vi "8bit sync-Gen patches montage B.vi"(0 "U8 Image (Montage)":T3, 1 "max value":dbl, 4 "Cycle number":i32, 5 "error in (no error)":errorcluster, 6 "Coordinates of montage positions":cluster{"X\n\nY":i32[]}[](array[cluster]), 8 "Extracted patches AVIs refs":T1[](array[typedef]), 9 "Frames info":T4, 11 "Image refs cluster":T2) -> (16 "U8 Image (Montage)":T3, 19 "error out":errorcluster)   [LabVIEW 2020]
uses:
  <vilib>/vision/Image Controls.llb/IMAQ Image.ctl
  Typedefs/8bit sync-IMAQ image refs.ctl
  <vilib>/vision/Avi.llb/IMAQ AVI2 Refnum.ctl
  Globals/gl_8-bit montage window ctrl refs.vi
  <vilib>/vision/NI_Vision_Development_Module.lvlib
panel:
  out "max value 3":u8
  out "max value 2":dbl
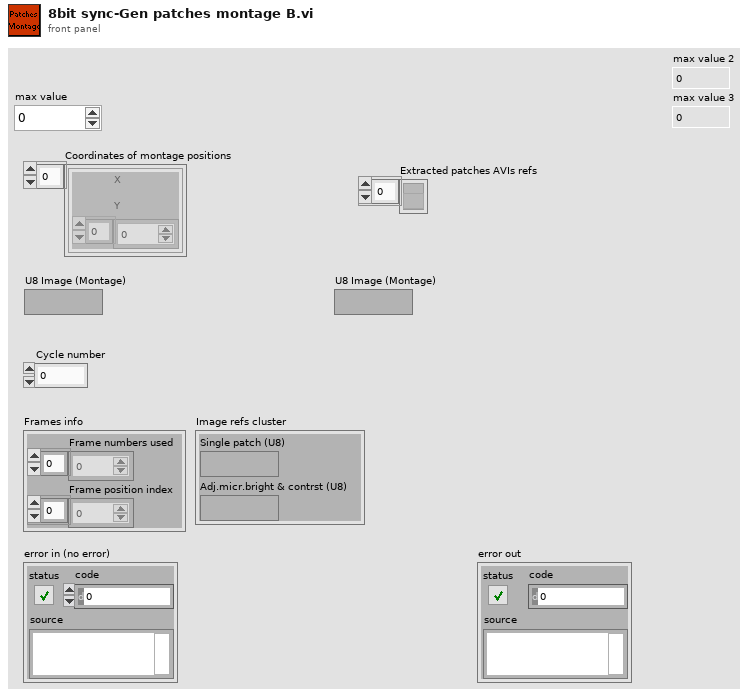
[diagram p1: front panel]
types:
  T1 = typedef "IMAQ AVI2 Refnum.ctl" = refnum<k20>
  T2 = typedef "8bit sync-IMAQ image refs.ctl" = cluster{"Single patch (U8)":T3, "Adj.micr.bright & contrst (U8)":T3}
  T3 = typedef "IMAQ Image.ctl" = refnum<image>
  T4 = cluster{"Frame numbers used":i32[], "Frame position index":i32[]}
  T5 = typedef "Image Type" = u32
  T6 = typedef "8-bit video export window ctrl refs.ctl" = cluster{"This VI":refnum<vi>, "Add speed data":refnum<vi>, "Add camera videos":refnum<vi>, "Stop button":refnum<vi>, "Camera Video Adjustments":refnum<vi>, "Microscope Image Adjustments":refnum<vi>, "Execute":refnum<vi>, "Codec":refnum<vi>, "Channel to load":refnum<vi>, "Speed graph behaviour":refnum<vi>, "Include speed graph":refnum<vi>, "Number of rows to generate":refnum<vi>, "Path":refnum<vi>}
  T7 = typedef "Bright-Contr-Gamma cluster.ctl" = cluster{"Brightness":sgl, "Contrast":sgl, "Gamma":sgl}
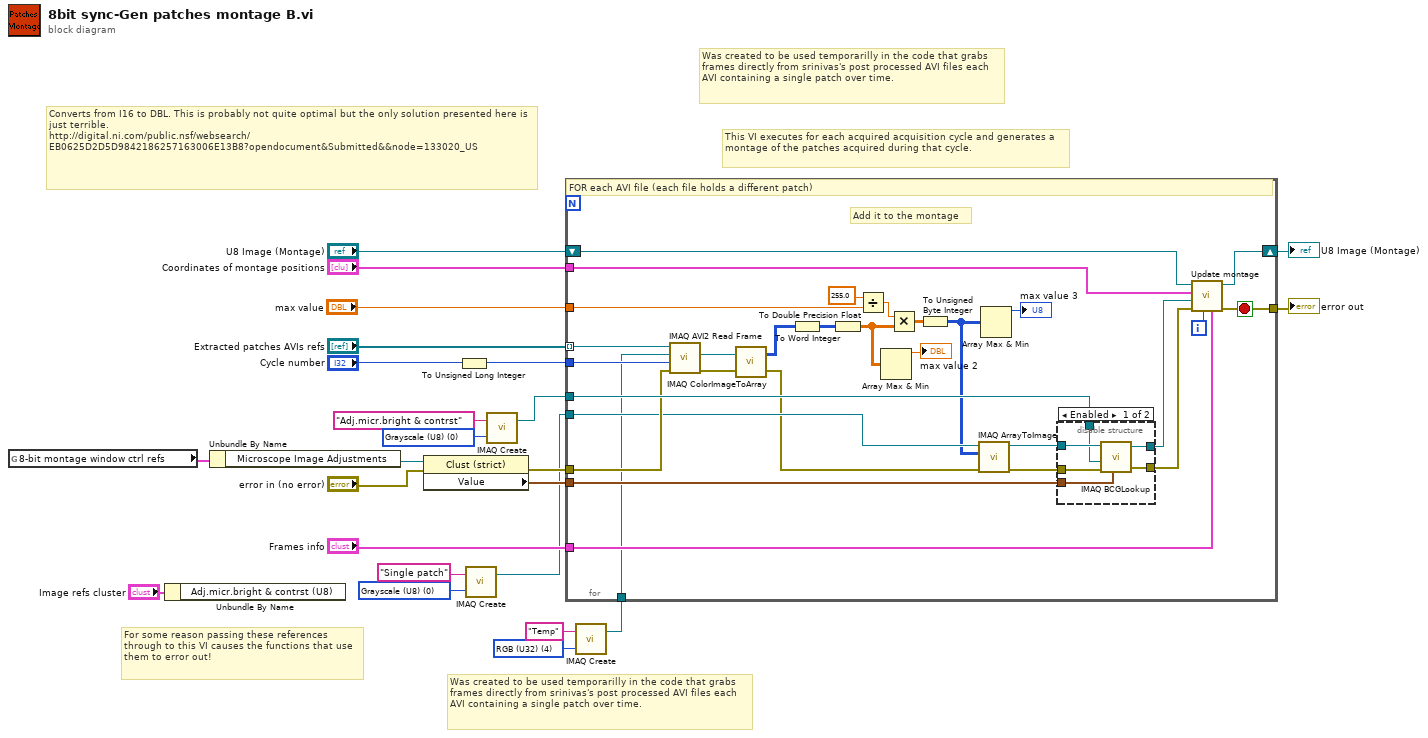
[diagram p0: block diagram]
diagram:
  w3 = T5 0 items=["Grayscale (U8)", "Grayscale (I16)", "Grayscale (SGL)", "Complex (CSG)", "RGB (U32)", "HSL (U32)", "RGB (U64)", "Grayscale (U16)"] ("Image Type")
  w6 = T5 0 items=["Grayscale (U8)", "Grayscale (I16)", "Grayscale (SGL)", "Complex (CSG)", "RGB (U32)", "HSL (U32)", "RGB (U64)", "Grayscale (U16)"] ("Image Type")
  w8 = T5 4 items=["Grayscale (U8)", "Grayscale (I16)", "Grayscale (SGL)", "Complex (CSG)", "RGB (U32)", "HSL (U32)", "RGB (U64)", "Grayscale (U16)"] ("Image Type")
  # "For some reason passing these references through to this VI causes the functions that use them to error out!"
  # "Was created to be used temporarilly in the code that grabs frames directly from srinivas's post processed AVI files each AVI containing a single patch over time."
  # "Was created to be used temporarilly in the code that grabs frames directly from srinivas's post processed AVI files each AVI containing a single patch over time."
  # "Converts from I16 to DBL. This is probably not quite optimal but the only solution presented here is just terrible.\nhttp://digital.ni.com/public.nsf/websearch/EB0625D2D5D9842186257163006E13B8?opendocument&Submitted&&node=133020_US"
  # "This VI executes for each acquired acquisition cycle and generates a montage of the patches acquired during that cycle."
  n1 = global read "gl_8-bit montage window ctrl refs.vi" "8-bit montage window ctrl refs"() -> (w18:T6)
  n2 = Unbundle By Name("Image refs cluster") -> ()  [unwired: 1 out]
  n3 = Unbundle By Name(w18) -> ("Microscope Image Adjustments"=w19:refnum<vi>)
  n4 = property class="Clust (strict)"(reference=w19, error in="error in (no error)") -> (error out=w15:errorcluster, "Value"=w16:T7)  [unwired: 1 out]
  n5 = To Unsigned Long Integer(number="Cycle number") -> (unsigned 32bit integer=w13:u32)
  n6 = call "IMAQ Create"("Image Name"="Single patch", "Image Type"=w6) -> ("New Image"=w2:T3)  [unwired: 2 in, 2 out]
  n7 = call "IMAQ Create"("Image Name"="Adj.micr.bright & contrst", "Image Type"=w3) -> ("New Image"=w1:T3)  [unwired: 3 in, 1 out]
  n8 = call "IMAQ Create"("Image Name"="Temp", "Image Type"=w8) -> ("New Image"=w7:T3)  [unwired: 3 in, 1 out]
  n9 = for {
    tunnel: [w49] -> w24
    tunnel: w15 -> [w43]
    shift-right: [w50] -> w23
    shift-left: "U8 Image (Montage)" -> [w54]
    tunnel: "Coordinates of montage positions" -> [w53]
    tunnel: "Frames info" -> [w51]
    tunnel: w16 -> [w46]
    tunnel: w1 -> [w45]
    tunnel: w13 -> [w44]
    tunnel: "max value" -> [w36]
    tunnel: w2 -> [w33]
    tunnel: "Extracted patches AVIs refs" -> [w31] mode=indexing
    tunnel: w7 -> [w30]
    i -> [w52]
    stop <- w49 stop-if-true
    # "Add it to the montage"
    # "FOR each AVI file (each file holds a different patch)"
    n10 = call "IMAQ AVI2 Read Frame"("error in (no error)"=w43, "Frame Number"=w44, "Image"=w30, "AVI Refnum"=w31) -> ("error out"=w32:errorcluster, "Image Out"=w42:T3)  [unwired: 5 in, 1 out]
    n11 = call "IMAQ ColorImageToArray"("Image"=w42, "error in (no error)"=w32) -> ("Image Pixels (U32)"=w35:u32[][], "error out"=w29:errorcluster)  [unwired: 1 in, 2 out]
    n12 = To Word Integer(number=w35) -> (16bit integer=w40:i16[][])
    n13 = To Double Precision Float(number=w40) -> (double precision float=w27:dbl[][])
    n14 = Divide(x=255.0 ("Numeric"), y=w36) -> (x/y=w38:dbl)
    n15 = Array Max & Min(array=w27) -> (max value=→"max value 2":dbl)  [unwired: 3 out]
    n16 = Multiply(x=w38, y=w27) -> (x*y=w39:dbl[][])
    n17 = To Unsigned Byte Integer(number=w39) -> (unsigned 8bit integer=w28:u8[][])
    n18 = call "IMAQ ArrayToImage"("error in (no error)"=w29, "Image Pixels (U8)"=w28, "Image"=w33) -> ("error out"=w34:errorcluster, "Image Out"=w41:T3)  [unwired: 7 in]
    n19 = Array Max & Min(array=w28) -> (max value=→"max value 3":u8)  [unwired: 3 out]
    n20 = disable-structure shown="Enabled" {
      disable-tunnel: [w60 w62] -> w48
      disable-tunnel: [w59 w61] -> w47
      disable-tunnel: w34 -> [w58 w61]
      disable-tunnel: w46 -> [w55 _]
      disable-tunnel: w41 -> [w57 w62]
      disable-tunnel: w45 -> [w56 _]
      frame Enabled {
        n21 = call "IMAQ BCGLookup"("Image Src"=w57, "BCG Values"=w55, "Image Dst"=w56, "error in (no error)"=w58) -> ("Image Dst Out"=w60:T3, "error out"=w59:errorcluster)  [unwired: 3 in]
      }
      frame Disabled {
      }
    }
    n22 = call "Update montage.vi"("Frames info"=w51, "Frame's rel. index"=w52, "Error in"=w47, "Single patch image"=w48, "Coordinates of montage positions"=w53, "Image (Montage)"=w54) -> ("error out"=w49:errorcluster, "Image (Montage)"=w50:T3)  [unwired: 4 in]
  }
  "error out" <- w24
  "U8 Image (Montage)" <- w23
